vi "main.vi"() -> ()   [LabVIEW 2010]
uses:
  common_typedefs/channels_cluster.ctl
  common_typedefs/gate_parameters_cluster.ctl
  OnBoardBuffer/OnBoardBuffer.ctl
  write-to-fifo_status.ctl
  <vilib>/Platform/TimedLoop/XDataNode/XDataNode.xnode
  <vilib>/Platform/TimedLoop/XDataNode/timing_clust.ctl
  <vilib>/Platform/TimedLoop/XDataNode/nitl_modes.ctl
  <vilib>/Platform/TimedLoop/XDataNode/wakeup.ctl
  <vilib>/eio/EIONode/EIONode.xnode
  <vilib>/rvi/eio/nirviEIOImplementation/nirviEIOImplementation.xnode
  <vilib>/rvi/eio/common/nirviEmuClasses.ctl
  <vilib>/rvi/DataTransferAndStorage/Container/XNode/niFpgaContainer.xnode
  <vilib>/rvi/eio/common/nirviEmuTemplateMethod_noerrors.vi
  <vilib>/rvi/FIFO/Fifo_Resource/nirvififoEmulationSetSize.vi
  <vilib>/rvi/DataTransferAndStorage/Container/Common/niFpgaContainerGetUniqueNameForEmu.vi
  <vilib>/Platform/TimedLoop/XDataNode/XDNodeRunTimeDep.lvlib
  OnBoardBuffer/OnBoardBuffer.lvlib
panel:
  in  "number of pixels":i64=-1
  in  "shall  acquisition start clocks?":bool
  in  "run clock 3":bool
  in  "run clock 2":bool
  in  "run clock 1":bool
  in  "clamp first pixel?":bool
  out "data received for buffering":u64
  out "local transfer FIFO full?":bool
  out "start acquisition?":bool
  out "write-to-FIFO status":T1
  out "on-board buffer":T2
  out "target-to-host FIFO full?":bool
  out "no. elements in on-board buffer":u32
  out "integration loop counter":i32
  in  "clock 3":T3
  in  "clock 2":T3
  in  "clock 1":T3
  out "integrated pixel values":T4
  out "data read":T4
  in  "channel offsets":T4
  out "clock 3 state":bool
  out "clock 2 state":bool
  out "clock 1 state":bool
  in  "wait for trigger?":bool
  in  "stop":bool
  in  "acquire":bool
  out "acquiring?":bool
  out "current pixel no.":i64
  in  "maximum bit depth":i8
  in  "iterations per pixel":u32
  # "Integration parameters"
  # "Outputs / displays"
  # "Clock parameters"
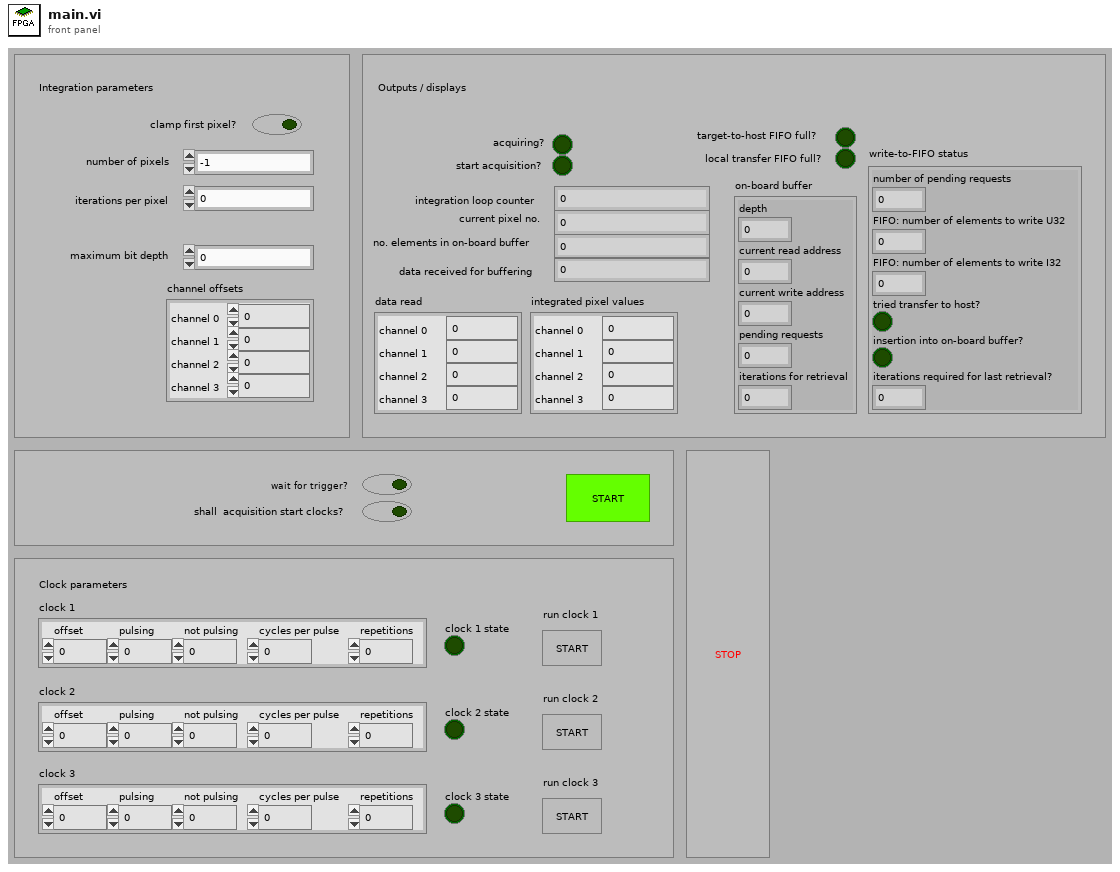
[diagram p1: front panel]
types:
  T1 = typedef "write-to-fifo_status.ctl" = cluster{"number of pending requests":i32, "FIFO: number of elements to write U32":u32, "FIFO: number of elements to write I32":i32, "tried transfer to host?":bool, "insertion into on-board buffer?":bool, "iterations required for last retrieval?":u32}
  T2 = typedef "OnBoardBuffer.lvlib/OnBoardBuffer.ctl" = cluster{"depth":u32, "current read address":u32, "current write address":u32, "pending requests":u32, "iterations for retrieval":u32}
  T3 = typedef "gate_parameters_cluster.ctl" = cluster{"offset":i64, "pulsing":i64, "not pulsing":i64, "cycles per pulse":i64, "repetitions":i64}
  T4 = typedef "channels_cluster.ctl" = cluster{"channel 0":u32, "channel 1":u32, "channel 2":u32, "channel 3":u32}
  T5 = typedef "XDNodeRunTimeDep.lvlib/timing_clust.ctl" = cluster{"Expected End [f-1]":u64, "Actual End [f-1]":u64, "Finished Late? [f-1]":bool, "Expected End [i-1]":u64, "Actual End [i-1]":u64, "Finished Late? [i-1]":bool, "Expected Start [i]":u64, "Actual Start [i]":u64, "Expected Start [f]":u64, "Actual Start [f]":u64, "Source Name":string, "Structure Name":string, "Period":i64, "Deadline":i64, "Offset":i64, "Start":i64, "Priority":i32, "Timeout":i32, "Mode":T6, "Wakeup Reason":T7, "Error":errorcluster, "Source Type":string, "Secondary Source Type":string, "Global End Time":u64, "Global Start Time":u64, "Frame Duration":u64, "Iteration Duration":u64, "Assigned CPU":i32, "I/O Scan Engine Mode":u32}
  T6 = typedef "XDNodeRunTimeDep.lvlib/nitl_modes.ctl" = enum32{"No Change", "Process missed periods, maintain original phase", "Discard missed periods, maintain original phase", "Process missed periods, ignore original phase", "Discard missed periods, ignore original phase"}
  T7 = typedef "XDNodeRunTimeDep.lvlib/wakeup.ctl" = enum32{"Normal", "Aborted", "Asynchronous wakeup", "Timing source error", "Timed loop error", "Timeout"}
  T8 = typedef "nirviEmuClasses.ctl" = enum16{"IO Read", "IO Write", "Method", "Property Read", "Property Write"}
  T9 = typedef "gate_counters_cluster.ctl" = cluster{"phase iteration counter":i64, "phase repetition counter":i64, "pulse iteration counter":i64, "phase state":bool}
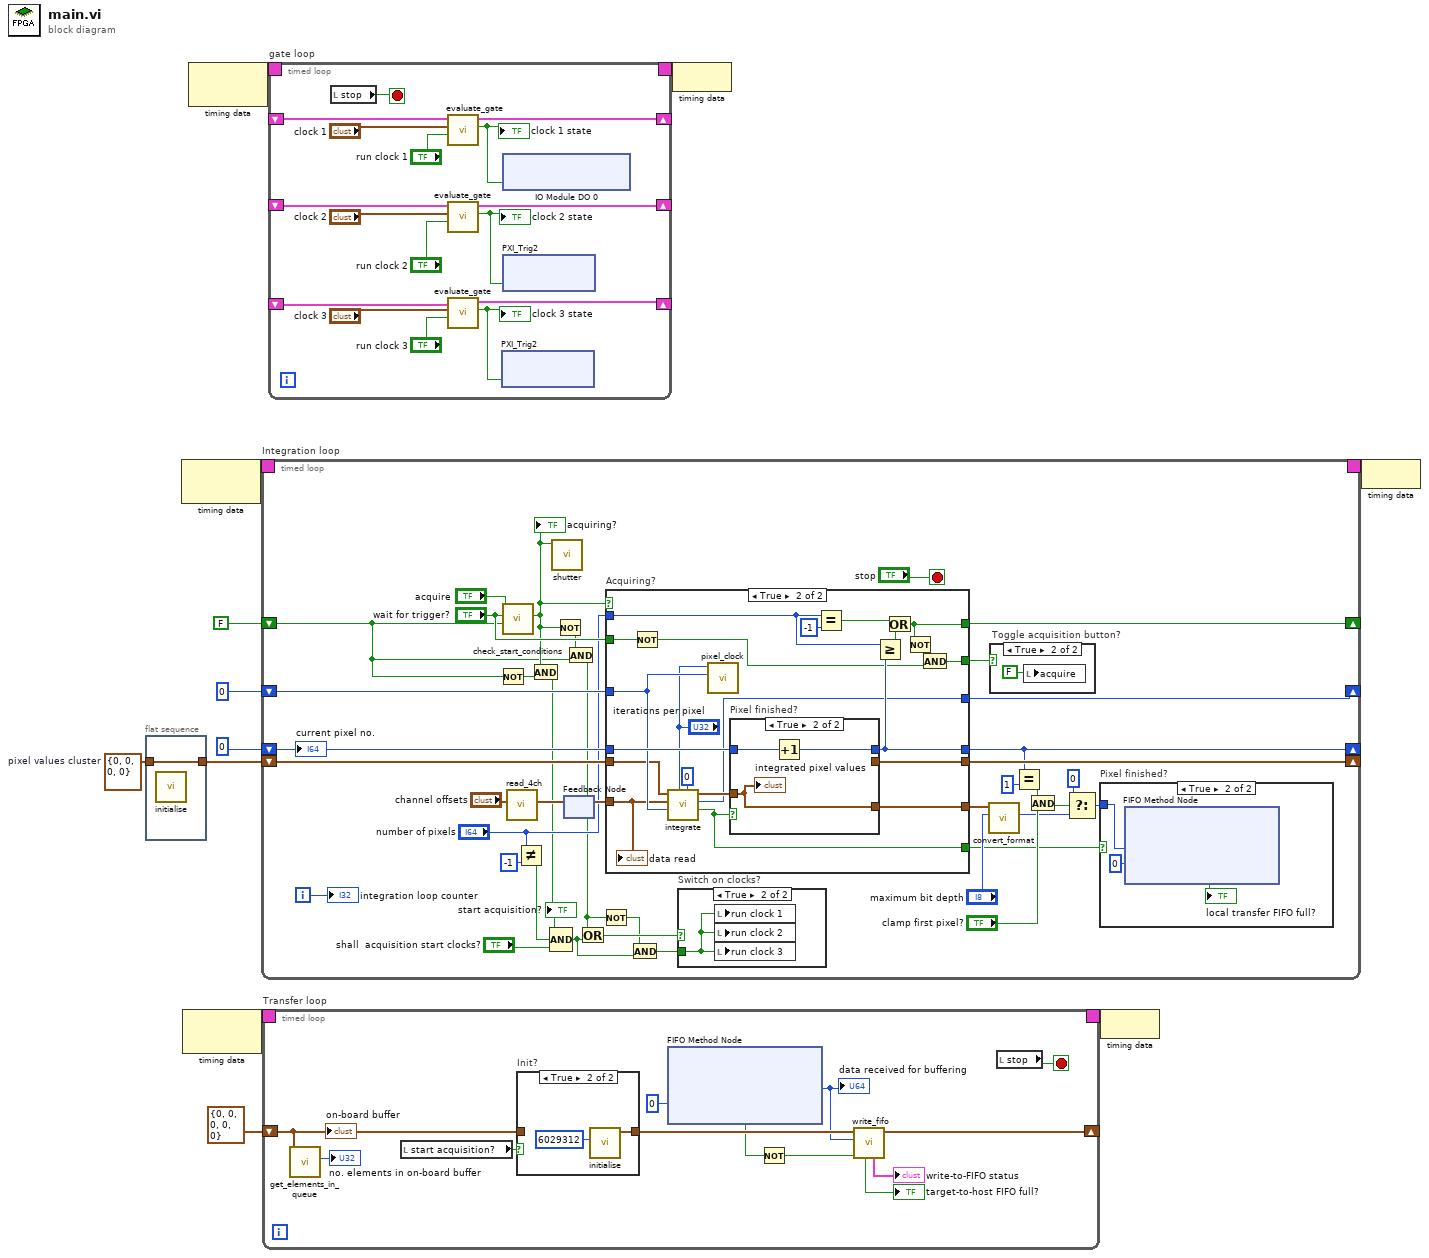
[diagram p0: block diagram]
diagram:
  w5 = T4 {"channel 0"=0, "channel 1"=0, "channel 2"=0, "channel 3"=0}  # pixel values cluster
  n1 = flat-sequence {
    tunnel: w5 -> [w13]
    tunnel: [w13] -> w4
    frame #0 {
      n2 = call "initialise.vi"() -> ()  [unwired: 12 in]
    }
  }
  n3 = node-c288() -> (w12:T5)  [unwired: 1 in]
  n4 = node-c288() -> (w2:T5)  [unwired: 1 in]
  n5 = node-c288() -> (w8:T5)  [unwired: 1 in]
  n6 = timed-loop "Integration loop" {
    timing: w12 -> [_]
    timing-out: [_] -> w11
    shift-right: [w32] -> _
    shift-left: i64 0 -> [w42]
    shift-right: [w47] -> _
    shift-left: u32 0 ("iteration counter out") -> [w49]
    shift-right: [w48] -> _
    shift-left: w4 -> [w50]
    shift-right: [w43] -> _
    shift-left: FALSE -> [w20]
    i -> [w39]
    stop <- "stop" stop-if-true
    n7 = Not(x=w20) -> (.not. x?=w38:bool)
    n8 = call "check_start_conditions.vi"("already acquiring?"=w20, "in triggered mode?"="wait for trigger?", "acquire"="acquire") -> ("acquire?"=w21:bool)  [unwired: 8 in]
    "acquiring?" <- w21
    n9 = call "read_4ch.vi"("channel offsets"="channel offsets") -> ("read output"=w45:T4)  [unwired: 10 in]
    n10 = Not Equal?(x="number of pixels", y=i64 -1 ("x")) -> (x != y?=w23:bool)
    n11 = And(x=w21, y=w38) -> (x .and. y?=w22:bool)
    "start acquisition?" <- w22
    n12 = Compound Arithmetic op=AND(w22, w23, "shall  acquisition start clocks?") -> (w16:bool)
    n13 = call "shutter.vi"("open?"=w21) -> ()  [unwired: 11 in]
    n14 = Not(x=w21) -> (.not. x?=w19:bool)
    n15 = feedback-in #1(w45) -> ()
    n16 = feedback #1() -> (w44:T4)  [unwired: 1 in]
    n17 = And(x=w19, y=w20) -> (x .and. y?=w17:bool)
    n18 = Or(x=w17, y=w16) -> (x .or. y?=w18:bool)
    n19 = Not(x=w17) -> (.not. x?=w15:bool)
    n20 = case "Acquiring?" shown="True" w21 {
      tunnel: [_ w116] -> w37
      tunnel: [_ w122] -> w47
      tunnel: [_ w126] -> w32
      tunnel: w50 -> [_ w119]
      tunnel: w42 -> [_ w124]
      tunnel: w49 -> [_ w121]
      tunnel: [_ w125] -> w48
      tunnel: w44 -> [_ w120]
      tunnel: [_ w115] -> w43
      tunnel: [_ w112] -> w40
      tunnel: "wait for trigger?" -> [_ w114]
      tunnel: [_ w110] -> w34
      tunnel: "number of pixels" -> [_ w109]
      frame False {
      }
      frame True {
        n21 = Not(x=w114) -> (.not. x?=w111:bool)
        n22 = call "integrate.vi"("waiting iterations per pixel"=u32 0, "integration iterations per pixel"="iterations per pixel", "iteration counter in"=w121, "sampling values in"=w120, "previous pixel values in"=w119) -> ("finished?"=w110:bool, "iteration counter out"=w122:u32, "new pixel values out"=w123:T4)  [unwired: 4 in]
        n23 = call "pixel_clock.vi"("current iteration"=w121, "iterations per pixel"="iterations per pixel") -> ()  [unwired: 10 in]
        n24 = case "Pixel finished?" shown="True" w110 {
          tunnel: w123 -> [w131 w134]
          tunnel: [_ w134] -> w116
          tunnel: [w130 w132] -> w126
          tunnel: w124 -> [w130 w133]
          tunnel: [w131 _] -> w125
          frame False {
          }
          frame True {
            n25 = Increment(x=w133) -> (x+1=w132:i64)
            "integrated pixel values" <- w134
          }
        }
        n26 = Equal?(x=w109, y=i64 -1 ("x")) -> (x = y?=w129:bool)
        n27 = Greater Or Equal?(x=w109, y=w126) -> (x >= y?=w128:bool)
        n28 = Or(x=w129, y=w128) -> (x .or. y?=w115:bool)
        n29 = Not(x=w115) -> (.not. x?=w113:bool)
        n30 = And(x=w113, y=w111) -> (x .and. y?=w112:bool)
        "data read" <- w120
      }
    }
    n31 = And(x=w15, y=w16) -> (x .and. y?=w14:bool)
    n32 = case "Switch on clocks?" shown="True" w18 {
      tunnel: w14 -> [_ w53]
      frame False {
      }
      frame True {
        n33 = local write "run clock 1"(w53) -> ()
        n34 = local write "run clock 2"(w53) -> ()
        n35 = local write "run clock 3"(w53) -> ()
      }
    }
    n36 = call "convert_format.vi"("maximum bit depth"="maximum bit depth", "values to be written"=w37) -> ("data"=w29:u64)  [unwired: 9 in]
    n37 = case "Toggle acquisition button?" shown="True" w40 {
      frame False {
      }
      frame True {
        n38 = local write "acquire"(FALSE) -> ()
      }
    }
    n39 = Equal?(x=w32, y=i64 1) -> (x = y?=w30:bool)
    n40 = And(x=w30, y="clamp first pixel?") -> (x .and. y?=w33:bool)
    n41 = Select(t=u64 0, s=w33, f=w29) -> (s? t:f=w28:u64)
    n42 = case "Pixel finished?" shown="True" w34 {
      tunnel: w28 -> [_ w56]
      frame False {
      }
      frame True {
        n43 = xnode ("FIFO Method Node")("Element"=w56, "Timeout"=0) -> ("Timed Out?"=→"local transfer FIFO full?":bool)  [unwired: 1 in, 1 out]
      }
    }
    "current pixel no." <- w42
    "integration loop counter" <- w39
  }
  n44 = timed-loop "Transfer loop" {
    shift-right: [w144] -> _
    shift-left: T2 {"depth"=0, "current read address"=0, "current write address"=0, "pending requests"=0, "iterations for retrieval"=0} ("on-board buffer out") -> [w147]
    timing: w2 -> [_]
    timing-out: [_] -> w1
    stop <- w142 stop-if-true
    n45 = call "get_elements_in_queue.vi"("on-board buffer in"=w147) -> ("no. elements"=→"no. elements in on-board buffer":u32)  [unwired: 10 in]
    n46 = local read "start acquisition?"() -> (w146:bool)
    n47 = case "Init?" shown="True" w146 {
      tunnel: [w200 w202] -> w145
      tunnel: w147 -> [w200 _]
      frame False {
      }
      frame True {
        n48 = call "initialise.vi"("depth"=u32 6029312) -> ("on-board buffer out"=w202:T2)  [unwired: 10 in]
      }
    }
    n49 = xnode ("FIFO Method Node")("Timeout"=0) -> ("Element"=w141:u64, "Timed Out?"=w138:bool)  [unwired: 1 in, 1 out]
    "data received for buffering" <- w141
    n50 = Not(x=w138) -> (.not. x?=w137:bool)
    n51 = call "write_fifo.vi"("input ready?"=w137, "data"=w141, "on-board buffer in"=w145) -> ("on-board buffer out"=w144:T2, "write-to-FIFO status"=→"write-to-FIFO status":T1, "FIFO full?"=→"target-to-host FIFO full?":bool)  [unwired: 6 in]
    n52 = local read "stop"() -> (w142:bool)
    "on-board buffer" <- w147
  }
  n53 = timed-loop "gate loop" {
    timing: w8 -> [_]
    timing-out: [_] -> w7
    shift-right: [w219] -> _
    shift-left: _ -> [w220]
    shift-right: [w217] -> _
    shift-left: _ -> [w218]
    shift-right: [w216] -> _
    shift-left: _ -> [w215]
    stop <- w211 stop-if-true
    n54 = local read "stop"() -> (w211:bool)
    n55 = call "evaluate_gate.vi"("acquiring?"="run clock 1", "gate settings"="clock 1", "gate counters in"=w220) -> ("pulse state out"=w205:bool, "gate counters out"=w219:T9)  [unwired: 7 in]
    "clock 1 state" <- w205
    n56 = call "evaluate_gate.vi"("acquiring?"="run clock 2", "gate settings"="clock 2", "gate counters in"=w218) -> ("pulse state out"=w207:bool, "gate counters out"=w217:T9)  [unwired: 7 in]
    "clock 2 state" <- w207
    n57 = call "evaluate_gate.vi"("acquiring?"="run clock 3", "gate settings"="clock 3", "gate counters in"=w215) -> ("pulse state out"=w206:bool, "gate counters out"=w216:T9)  [unwired: 7 in]
    "clock 3 state" <- w206
    n58 = xnode "PXI_Trig2"("PXI_Trig2"=w206) -> ()  [unwired: 1 in, 1 out]
    n59 = xnode "IO Module DO 0"("IO Module\\D0 0"=w205) -> ()  [unwired: 1 in, 1 out]
    n60 = xnode "PXI_Trig2"("PXI_Trig1"=w207) -> ()  [unwired: 1 in, 1 out]
  }
  n61 = node-c288(w7) -> ()
  n62 = node-c288(w1) -> ()
  n63 = node-c288(w11) -> ()
